vi "Accessor - Set.vi"(8 "error in (no error)":errorcluster, 9 "values":variant[](array[variant]), 10 "keys":string[](array[string]), 11 "uData in":refnum<class "uData.lvclass">) -> (0 "error out":errorcluster, 3 "uData out":refnum<class "uData.lvclass">, 4 "replaced?":bool[](array[boolean]))   [LabVIEW 2023, in "uLib.lvlib" / "uData.lvclass"]
doc: "This is a (SET) accessor to use by all other methods. It performs key conditioning, array size match check and calls the dynamic dispatch inline operation. It handles output values on error as well."
uses:
  uData.lvclass
  uData.lvclass/uData.ctl
  Condition Tag Name.vi
  Blank Key Reserved String.vi
  <vilib>/Utility/error.llb/Error Cluster From Error Code.vi
  <vilib>/ErrorRing/Error Ring.xnode
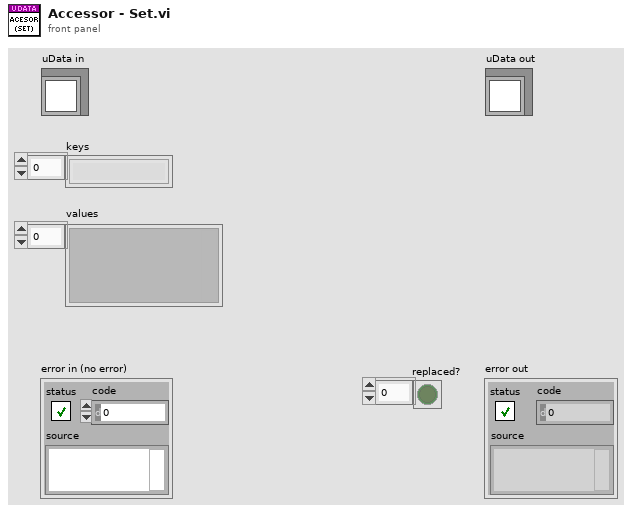
[diagram p1: front panel]
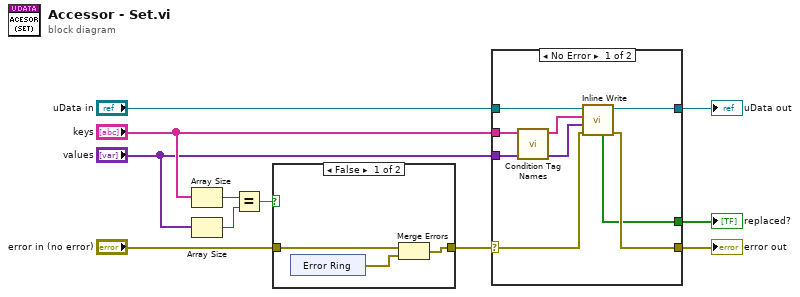
[diagram p0: block diagram]
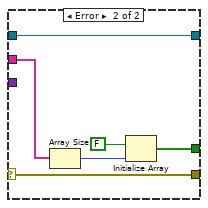
[diagram p2: hidden frame]
diagram:
  n1 = Array Size(array="keys") -> (size(s)=w5:i32)
  n2 = Array Size(array="values") -> (size(s)=w4:i32)
  n3 = Equal?(x=w5, y=w4) -> (x = y?=w3:bool)
  n4 = case shown="False" w3 {
    tunnel: "error in (no error)" -> [w13 w20]
    tunnel: [w14 w20] -> w1
    frame False {
      n5 = xnode "Error Ring"() -> ("error out"=w12:errorcluster)
      n6 = Merge Errors(w13, w12) -> (w14:errorcluster)
    }
    frame True {
    }
  }
  n7 = case shown="No Error" w1 {
    selector: w1 -> [w26 w34]
    tunnel: [w25 w34] -> w11
    tunnel: [w28 w33] -> w9
    tunnel: "uData in" -> [w27 w33]
    tunnel: [w24 w29] -> w8
    tunnel: "values" -> [w23 _]
    tunnel: "keys" -> [w22 w30]
    frame No Error {
      n8 = call "Condition Tag Names.vi"("tags in"=w22) -> ("tags out"=w21:string[])  [unwired: 10 in]
      n9 = call "Inline Write.vi"("error in (no error)"=w26, "values"=w23, "keys"=w21, "uData in"=w27) -> ("error out"=w25:errorcluster, "uData out"=w28:refnum<class "uData.lvclass">, "replaced?"=w24:bool[])  [unwired: 5 in]
    }
    frame Error {
      n10 = Array Size(array=w30) -> (size(s)=w32:i32)
      n11 = Initialize Array(FALSE, w32) -> (w29:bool[])
    }
  }
  "error out" <- w11
  "uData out" <- w9
  "replaced?" <- w8
